vi "update status.vi"(9 "read messages from AUV sparus in":T1, 10 "Subtask registered event in":T2[][](array[typedef])) -> (0 "zmiana statusu  nadawanaego do robota lub komunikatu do robota":bool, 2 "read messages from AUV sparus out":T1, 3 "Subtask registered event out":T2[][](array[typedef]))   [LabVIEW 2015, in "Biblioteka moduł map v3.lvlib" / "task erl.lvlib"]
uses:
  TASK ERL/task erl.lvlib
  TASK ERL/List of robots.ctl
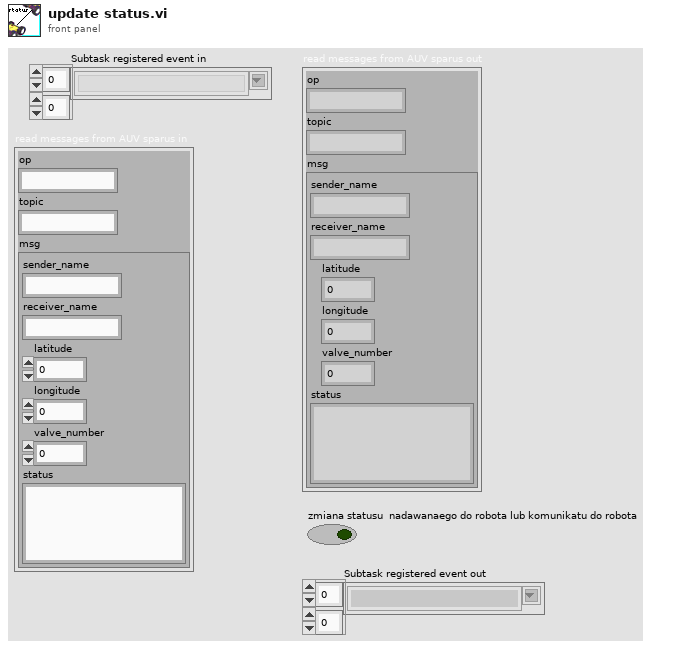
[diagram p1: front panel]
types:
  T1 = cluster{"op":string, "topic":string, "msg":cluster{"sender_name":string, "receiver_name":string, "latitude":dbl, "longitude":dbl, "valve_number":i32, "status":string}}
  T2 = typedef "Biblioteka moduł map v3.lvlib/task erl.lvlib/List of robots.ctl" = string
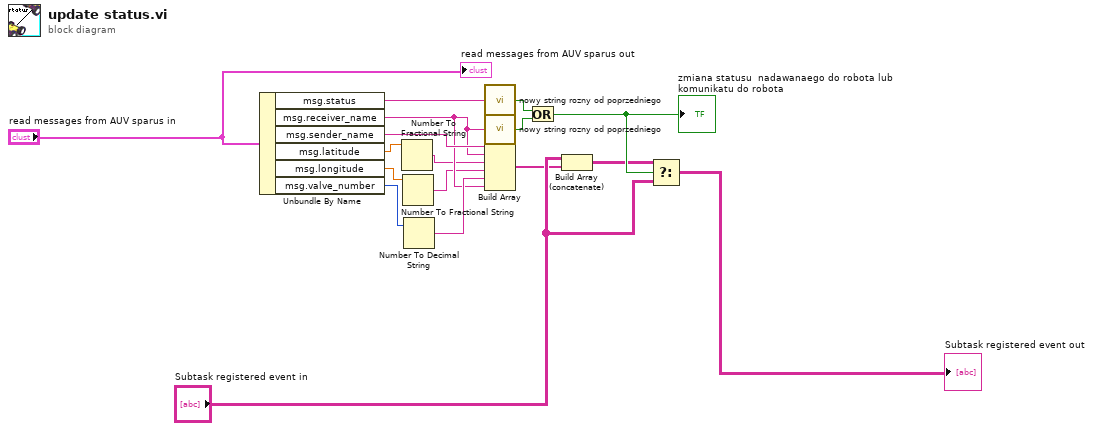
[diagram p0: block diagram]
diagram:
  n1 = Unbundle By Name("read messages from AUV sparus in") -> ("msg.status"=w10:string, "msg.receiver_name"=w6:string, "msg.sender_name"=w7:string, "msg.latitude"=w5:dbl, "msg.longitude"=w3:dbl, "msg.valve_number"=w11:i32)
  n2 = Number To Fractional String(number=w5) -> (F-format string=w4:string)  [unwired: 3 in]
  n3 = Number To Fractional String(number=w3) -> (F-format string=w2:string)  [unwired: 3 in]
  n4 = Number To Decimal String(number=w11) -> (decimal integer string=w12:string)  [unwired: 1 in]
  n5 = call "nowy string rozny od poprzedniego.vi"("String"=w10) -> ("x != y?"=w9:bool)  [unwired: 4 in]
  n6 = call "nowy string rozny od poprzedniego.vi"("String"=w6) -> ("x != y?"=w8:bool)  [unwired: 4 in]
  n7 = Build Array(w7, w6, w4, w2, w12, w6) -> (w13:string[])
  n8 = Or(x=w9, y=w8) -> (x .or. y?=w17:bool)
  "zmiana statusu  nadawanaego do robota lub komunikatu do robota" <- w17
  n9 = Build Array (concatenate)("Subtask registered event in", w13) -> (w14:T2[][])
  n10 = Select(t=w14, s=w17, f="Subtask registered event in") -> (s? t:f=→"Subtask registered event out":T2[][])
  "read messages from AUV sparus out" <- "read messages from AUV sparus in"
